vi "SaveExtract.vi"(8 "error in (no error)":errorcluster, 11 "VisionUI in":refnum<class "VisionUI.lvclass">) -> (0 "error out":errorcluster, 3 "VisionUI out":refnum<class "VisionUI.lvclass">)   [LabVIEW 2021, in "VisionUI.lvlib" / "VisionUI.lvclass"]
uses:
  VisionUI.lvclass
  C:/Users/alan0/Desktop/WebSocket/Actors/Vision/Vision/Vision.lvclass
  VisionUI.lvclass/VisionUI.ctl
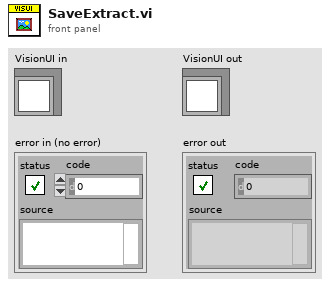
[diagram p1: front panel]
types:
  T1 = typedef "IMAQ Image.ctl" = refnum<image>
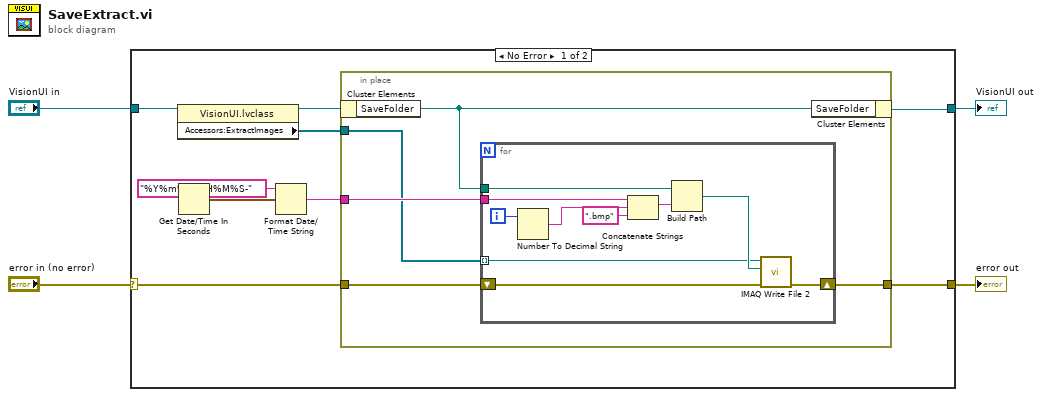
[diagram p0: block diagram]
diagram:
  n1 = case shown="No Error" "error in (no error)" {
    selector: "error in (no error)" -> [w6 w30]
    tunnel: [w5 w30] -> w3
    tunnel: [w11 w29] -> w1
    tunnel: "VisionUI in" -> [w13 w29]
    frame No Error {
      n2 = property class="VisionUI.lvclass"(reference=w13) -> (reference out=w12:refnum<class "VisionUI.lvclass">, "Accessors:ExtractImages"=w7:T1[])  [unwired: 1 in, 1 out]
      n3 = Get Date/Time In Seconds() -> (seconds since 1Jan1904=w10:timestamp)
      n4 = Format Date/Time String(time format string (%c)="%Y%m%d_%H%M%S-", seconds (now)=w10) -> (date/time string=w8:string)  [unwired: 1 in]
      n5 = in-place {
        in-place-border: w8 -> [w17]
        in-place-border: w7 -> [w16]
        in-place-border: w6 -> [w15]
        in-place-border: [w14] -> w5
        n6 = in-place-cluster #1(w12) -> ("SaveFolder"=w18:path)
        n7 = for {
          tunnel: w18 -> [w28]
          tunnel: w17 -> [w26]
          tunnel: w16 -> [w22] mode=indexing
          shift-right: [w20] -> w14
          shift-left: w15 -> [w21]
          i -> [w27]
          n8 = Number To Decimal String(number=w27) -> (decimal integer string=w25:string)  [unwired: 1 in]
          n9 = Concatenate Strings(w26, w25, ".bmp" ("string")) -> (w24:string)
          n10 = Build Path(base path=w28, name or relative path=w24) -> (appended path=w23:path)
          n11 = call-poly "IMAQ Write File 2"("error in (no error)"=w21, "File Path"=w23, "Image"=w22) -> ("error out"=w20:errorcluster)  [unwired: 7 in, 1 out]
        }
        n12 = in-place-cluster #1("SaveFolder"=w18) -> (w11:refnum<class "VisionUI.lvclass">)
      }
    }
    frame Error {
    }
  }
  "error out" <- w3
  "VisionUI out" <- w1
